vi "StopGlobal.vi"() -> ()   [LabVIEW 2013, in "Nav6.lvlib"]
uses:
  Nav6.lvlib
panel:
  in  "Stop":bool
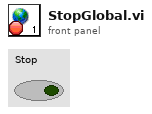
[diagram p1: front panel]
diagram:
